vi "CallEngine.vi"(8 "error in (no error)":errorcluster, 10 "RT_Game.lvlib:Engine.lvclass":refnum<class "Engine.lvclass">, 11 "Menu in":refnum<class "Menu.lvclass">) -> (0 "error out":errorcluster, 2 "RT_Game.lvlib:Engine.lvclass 2":refnum<class "Engine.lvclass">, 3 "Menu out":refnum<class "Menu.lvclass">)   [LabVIEW 2019, in "RT_Game.lvlib" / "Menu.lvclass"]
uses:
  Menu.lvclass
  Engine/Engine.lvclass
  Engine/Engine.lvclass/Engine.ctl
  Engine/Write delta_t.vi
  Game/Game.lvclass
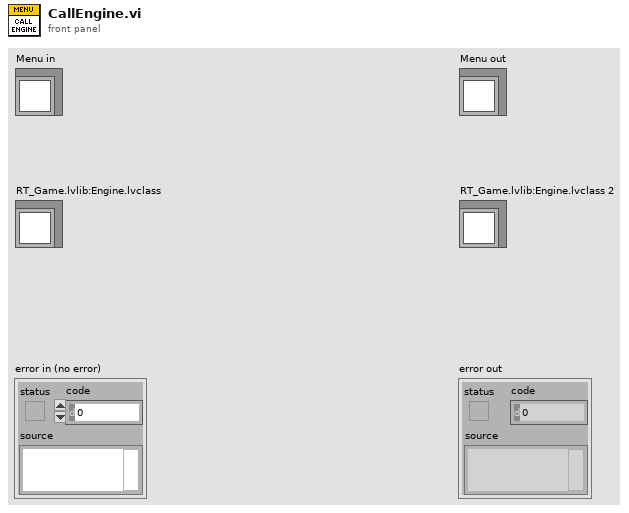
[diagram p1: front panel]
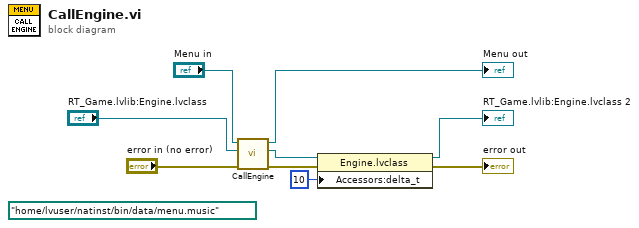
[diagram p0: block diagram]
diagram:
  (unwired) path "/home/lvuser/natinst/bin/data/menu.music" ("Path")
  n1 = call-parent "CallEngine.vi"("error in (no error)"="error in (no error)", "RT_Game.lvlib:Engine.lvclass"="RT_Game.lvlib:Engine.lvclass", "Game in"="Menu in") -> ("error out"=w9:errorcluster, "RT_Game.lvlib:Engine.lvclass 2"=w3:refnum<class "Engine.lvclass">, "Game out"=→"Menu out":refnum<class "Menu.lvclass">)  [unwired: 6 in]
  n2 = property class="Engine.lvclass"(reference=w3, error in=w9, "Accessors:delta_t"=u16 10 ("delta_t")) -> (reference out=→"RT_Game.lvlib:Engine.lvclass 2":refnum<class "Engine.lvclass">, error out=→"error out":errorcluster)
